vi "Refresh Status.vi"(8 "error in":errorcluster, 11 "PowerSupply in":refnum<class "PowerSupply.lvclass">) -> (0 "error out":errorcluster, 3 "PowerSupply out":refnum<class "PowerSupply.lvclass">)   [LabVIEW 2019, in "PowerSupply.lvlib" / "PowerSupply.lvclass"]
uses:
  Library/PowerSupply.lvclass
  Library/PowerSupply.lvclass/PowerSupply.ctl
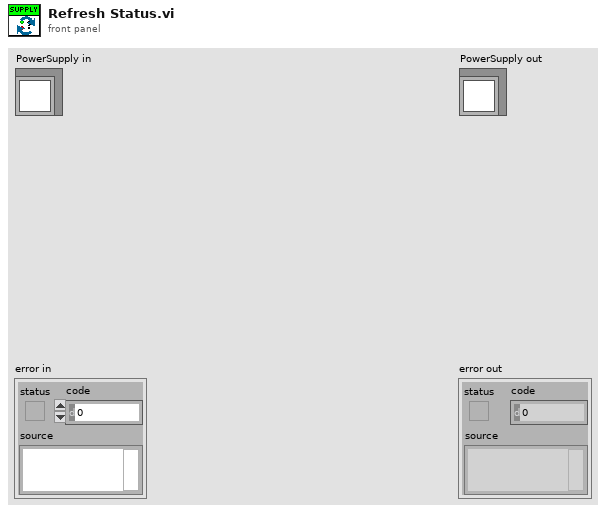
[diagram p1: front panel]
types:
  T1 = typedef "PowerSupply.lvlib/PowerSupply.lvclass/Status_Flags.ctl" = cluster{"Interlock":bool, "OVP":bool, "OCP":bool, "Output":bool}
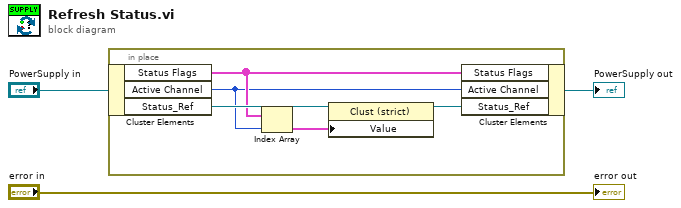
[diagram p0: block diagram]
diagram:
  n1 = in-place {
    n2 = in-place-cluster #1("PowerSupply in") -> ("Status Flags"=w6:T1[], "Active Channel"=w5:u32, "Status_Ref"=w8:refnum<vi>)
    n3 = Index Array(array=w6, index=w5) -> (element=w4:T1)
    n4 = property class="Clust (strict)"(reference=w8, "Value"=w4) -> (reference out=w7:refnum<vi>)  [unwired: 1 in, 1 out]
    n5 = in-place-cluster #1("Status Flags"=w6, "Active Channel"=w5, "Status_Ref"=w7) -> (→"PowerSupply out":refnum<class "PowerSupply.lvclass">)
  }
  "error out" <- "error in"
